vi "LVFunction_Imop_Compute_GaussianParametersComplete.vi"(0 "HasoField in":refnum<class "HasoField.lvclass">, 5 "Path":path, 7 "ArrayOfPSF":refnum<class "SurfaceFloat.lvclass">[](array[class]), 11 "error in (no error)":errorcluster, 12 "degree":sgl, 13 "spottype":enum16{"square", "circle"}(ring)) -> (1 "Gaussian Param":T2, 2 "tab_max_energy":sgl[](array[numeric]), 3 "Data_ mm":T1, 4 "HasoField out":refnum<class "HasoField.lvclass">, 8 "ArrayOfPSF out":refnum<class "SurfaceFloat.lvclass">[](array[class]), 10 "threshold":sgl, 14 "threshold_validity":bool, 15 "error out":errorcluster)   [LabVIEW 2020]
doc: "Complete gaussian parameters function.\n\n--------------------------------------------------------------------------------\n\n<B>config_file_pathIn</B> : Absolute path to the Haso configuration file.\n\n<B>config_file_pathOut</B> : Absolute path to the Haso configuration file.\n\n<B>HasoField</B> : HasoField object.\n\n<B>nb_planes</B> : Number of planes.\n\n<B>waist_position_millimeter</B> : Waist position (mm).\n\n<B>waist_radius_millimeter</B> : Waist radius (mm).\n\n<B>rayleigh_length_millimeter</B> : Rayleigh length (mm).\n\n<B>divergence</B> : Mivergence of the beam.\n\n<B>msquared</B> : m squared parameter.\n\n<B>spot_type</B> : \"square\" or \"circle\" spot shape.\n\n<B>degree</B> : Angle of the square spot shape forms with an horizontal axis (degree).///<\n\n<B>tab_z_cote_mm</B> : Array of z cote (mm) of the different planes.\n\n<B>tab_spot_size_mm</B> : Array of spot size (mm) of the different planes.\n\n<B>tab_psf</B> : Array of computed psf.\n\n<B>threshold</B> : Check whether the entire beam of last processing could be got.\n\n<B>tab_max_energy</B> : Array of max energy of the different planes.\n\n<B>ErrorIn</B> : Error\n\n<B>ErrorOut</B> : Error"
uses:
  HasoField.lvclass
  SurfaceFloat.lvclass
  LVClasse_SurfaceFloat Read SurfaceFloat.vi
  LVClass_HasoField Read HasoField.vi
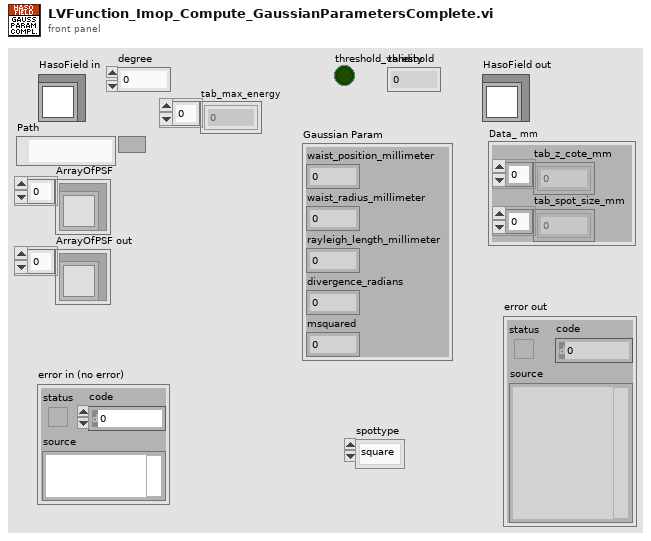
[diagram p1: front panel]
types:
  T1 = cluster{"tab_z_cote_mm":dbl[], "tab_spot_size_mm":dbl[]}
  T2 = cluster{"waist_position_millimeter":sgl, "waist_radius_millimeter":sgl, "rayleigh_length_millimeter":sgl, "divergence_radians":sgl, "msquared":sgl}
  T3 = typedef "ClassID.ctl" = i64
  T4 = cluster{"tab_z_cote_mm":sgl[], "tab_spot_size_mm":sgl[]}
  T5 = cluster{"waist_position_millimeter":sgl, "waist_radius_millimeter":sgl, "rayleigh_length_millimeter":sgl, "divergence":sgl, "msquared":sgl}
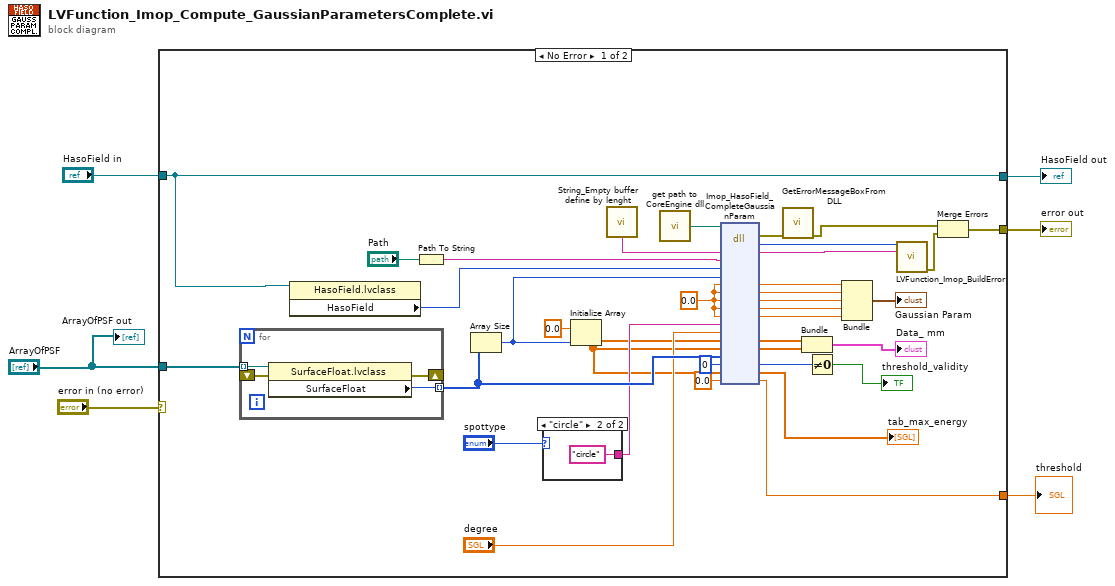
[diagram p0: block diagram]
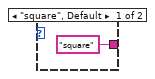
[diagram p2: hidden frame]
diagram:
  n1 = case shown="No Error" "error in (no error)" {
    selector: "error in (no error)" -> [_ w49]
    tunnel: "HasoField in" -> [w25 w50]
    tunnel: [w25 w50] -> w6
    tunnel: [w38 w49] -> w4
    tunnel: "ArrayOfPSF" -> [w19 _]
    tunnel: [w7 _] -> w1
    frame No Error {
      w32 = sgl 0.0 ("waist_position_millimeter")
      n2 = for {
        tunnel: w19 -> [w47] mode=indexing
        tunnel: [w48] -> w18 mode=indexing
        shift-right: [w45] -> _
        shift-left: _ -> [w46]
        n3 = property class="SurfaceFloat.lvclass"(reference=w47, error in=w46) -> (error out=w45:errorcluster, "SurfaceFloat"=w48:T3)  [unwired: 1 out]
      }
      n4 = property class="HasoField.lvclass"(reference=w25) -> ("HasoField"=w24:T3)  [unwired: 1 in, 2 out]
      n5 = Path To String(path="Path") -> (string=w33:string)
      n6 = Array Size(array=w18) -> (size(s)=w17:i32)
      n7 = case shown="\"circle\"" "spottype" {
        tunnel: ["square" "circle"] -> w14
        frame "square", Default {
        }
        frame "circle" {
        }
      }
      n8 = Initialize Array(0.0 ("element"), w17) -> (w10:dbl[])
      n9 = call "String_Empty buffer define by lenght.vi"() -> ("Empty buffer"=w37:string)  [unwired: 1 in]
      n10 = call "get path to CoreEngine dll.vi"() -> ("path to wavekit library"=w36:path)  [unwired: 14 in, 1 out]
      n11 = dll-call lib="D:/2_trunk/Soft_haso/ImOpCoreEngine4_LV2011/DLLs/ImopEngine4_vc100.dll" fn="Imop_HasoField_CompleteGaussianParam"(path in=w36, "message"=w37, "config file"=w33, "HasoField"=w24, "nb_planes"=w17, "waist_position_millimeter"=w32, "waist_radius_millimeter"=w32, "rayleigh_length_millimeter"=w32, "divergence"=w32, "msquared"=w32, "spottype"=w14, "degree"="degree", "tab_z_cote_mm"=w10, "tab_spot_size_mm"=w10, "tab_psf"=w18, "threshold_validity"=u8 0 ("threshold"), "tab_max_energy"=w10, "threshold"=sgl 0.0) -> (error out=w35:errorcluster, "return type"=w41:i32, "message"=w42:string, "waist_position_millimeter"=w31:sgl, "waist_radius_millimeter"=w30:sgl, "rayleigh_length_millimeter"=w29:sgl, "divergence"=w28:sgl, "msquared"=w27:sgl, "tab_z_cote_mm"=w23:sgl[], "tab_spot_size_mm"=w22:sgl[], "threshold_validity"=w12:u8, "tab_max_energy"=→"tab_max_energy":sgl[], "threshold"=w7:sgl)  [unwired: 8 in, 1 out]
      n12 = call "GetErrorMessageBoxFromDLL.vi"("error IN"=w35) -> ("error OUT"=w40:errorcluster)  [unwired: 10 in]
      n13 = Bundle("tab_z_cote_mm"=w23, "tab_spot_size_mm"=w22) -> (→"Data_ mm":T4)  [unwired: 1 in]
      n14 = Not Equal To 0?(x=w12) -> (x != 0?=→"threshold_validity":bool)
      n15 = Bundle("waist_position_millimeter"=w31, "waist_radius_millimeter"=w30, "rayleigh_length_millimeter"=w29, "divergence"=w28, "msquared"=w27) -> (→"Gaussian Param":T5)  [unwired: 1 in]
      n16 = call "LVFunction_Imop_BuildError.vi"("code"=w41, "String to Prepend to source (\"\")"=w42) -> ("error out"=w39:errorcluster)  [unwired: 13 in]
      n17 = Merge Errors(w40, w39) -> (w38:errorcluster)
    }
    frame Error {
    }
  }
  "error out" <- w4
  "HasoField out" <- w6
  "threshold" <- w1
  "ArrayOfPSF out" <- "ArrayOfPSF"
